vi "2 Channel Analog Output v1_0.vi"(1 "Voltage output 1":dbl(slide) scale=0.0..10.0, 2 "Voltage output 0":dbl(slide) scale=0.0..10.0) -> ()   [LabVIEW 2012]
uses:
  <vilib>/Utility/error.llb/DialogType.ctl
  <vilib>/DAQmx/write.llb/DAQmx Write (Analog 2D DBL NChan NSamp).vi
  <vilib>/DAQmx/create/channels.llb/DAQmx Create Channel (AO-Voltage-Basic).vi
  <vilib>/DAQmx/miscellaneous.llb/DAQmx Fill In Error Info.vi
panel:
  in  "minimum value":dbl=-10.0 format="%0.2f"
  in  "maximum value":dbl=10.0 format="%0.2f"
  in  "physical channels":tag="Dev1/ao0:1"
  # "This VI is able to talk to both Pumps at the same time.  It was simplified from the a previous version that was used in a Laptop Set-up. If the channel iis changed, just reinitialize values to default which is located under the Edit Drop down menu!"
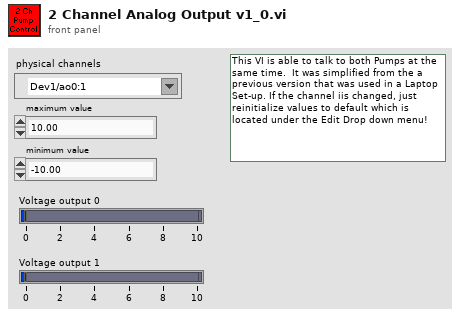
[diagram p1: front panel]
types:
  T1 = typedef "DialogType.ctl" = u16
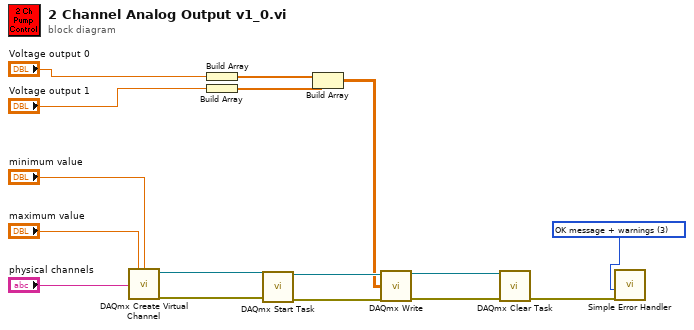
[diagram p0: block diagram]
diagram:
  w11 = T1 3 items=["no dialog", "OK message", "continue or stop message", "OK message + warnings", "continue/stop + warnings"] ("type of dialog (OK msg:1)")
  n1 = call-poly <vilib>:"DAQmx Create Virtual Channel.vi"("maximum value"="maximum value", "minimum value"="minimum value", "physical channels"="physical channels") -> ("task out"=w10:refnum<k21>, "error out"=w9:errorcluster)  [unwired: 11 in]
  n2 = Build Array("Voltage output 0") -> (w3:dbl[])
  n3 = Build Array("Voltage output 1") -> (w2:dbl[])
  n4 = call <vilib>:"DAQmx Start Task.vi"("task/channels in"=w10, "error in"=w9) -> ("task out"=w16:refnum<k21>, "error out"=w15:errorcluster)  [unwired: 12 in]
  n5 = Build Array(w3, w2) -> (w1:dbl[][])
  n6 = call-poly <vilib>:"DAQmx Write.vi"("task/channels in"=w16, "data"=w1, "error in"=w15) -> ("task out"=w14:refnum<k21>, "error out"=w13:errorcluster)  [unwired: 10 in, 1 out]
  n7 = call <vilib>:"DAQmx Clear Task.vi"("task in"=w14, "error in"=w13) -> ("error out"=w12:errorcluster)  [unwired: 13 in]
  n8 = call <vilib>:"Simple Error Handler.vi"("type of dialog (OK msg:1)"=w11, "error in (no error)"=w12) -> ()  [unwired: 3 in, 5 out]
